vi "OCV Histogram gRPC.vi"() -> (1 "mean values of channels":dbl[](array[numeric]), 2 "std dev":dbl, 3 "range":dbl)   [LabVIEW 2019] (continued)
"battery10voltage"=0.0, "battery11voltage"=0.0, "battery12voltage"=0.0, "battery13voltage"=0.0, "battery14voltage"=0.0, "battery15voltage"=0.0, "battery16voltage"=0.0, "battery17voltage"=0.0, "battery18voltage"=0.0, "battery19voltage"=0.0, "battery20voltage"=0.0, "battery21voltage"=0.0, "battery22voltage"=0.0, "battery23voltage"=0.0, "battery24voltage"=0.0, "ErrorOutData"={"ErrorCode"=0, "ErrorMessage"=""}}, {"battery1voltage"=3.481647, "battery2voltage"=3.483053, "battery3voltage"=3.4783683, "battery4voltage"=3.4823787, "battery5voltage"=3.484421, "battery6voltage"=0.0, "battery7voltage"=0.0, "battery8voltage"=0.0, "battery9voltage"=0.0, "battery10voltage"=0.0, "battery11voltage"=0.0, "battery12voltage"=0.0, "battery13voltage"=0.0, "battery14voltage"=0.0, "battery15voltage"=0.0, "battery16voltage"=0.0, "battery17voltage"=0.0, "battery18voltage"=0.0, "battery19voltage"=0.0, "battery20voltage"=0.0, "battery21voltage"=0.0, "battery22voltage"=0.0, "battery23voltage"=0.0, "battery24voltage"=0.0, "ErrorOutData"={"ErrorCode"=0, "ErrorMessage"=""}}, {"battery1voltage"=3.4816504, "battery2voltage"=3.4830518, "battery3voltage"=3.4783711, "battery4voltage"=3.4823825, "battery5voltage"=3.484416, "battery6voltage"=0.0, "battery7voltage"=0.0, "battery8voltage"=0.0, "battery9voltage"=0.0, "battery10voltage"=0.0, "battery11voltage"=0.0, "battery12voltage"=0.0, "battery13voltage"=0.0, "battery14voltage"=0.0, "battery15voltage"=0.0, "battery16voltage"=0.0, "battery17voltage"=0.0, "battery18voltage"=0.0, "battery19voltage"=0.0, "battery20voltage"=0.0, "battery21voltage"=0.0, "battery22voltage"=0.0, "battery23voltage"=0.0, "battery24voltage"=0.0, "ErrorOutData"={"ErrorCode"=0, "ErrorMessage"=""}}, {"battery1voltage"=3.4816463, "battery2voltage"=3.483057, "battery3voltage"=3.4783702, "battery4voltage"=3.4823778, "battery5voltage"=3.4844162, "battery6voltage"=0.0, "battery7voltage"=0.0, "battery8voltage"=0.0, "battery9voltage"=0.0, "battery10voltage"=0.0, "battery11voltage"=0.0, "battery12voltage"=0.0, "battery13voltage"=0.0, "battery14voltage"=0.0, "battery15voltage"=0.0, "battery16voltage"=0.0, "battery17voltage"=0.0, "battery18voltage"=0.0, "battery19voltage"=0.0, "battery20voltage"=0.0, "battery21voltage"=0.0, "battery22voltage"=0.0, "battery23voltage"=0.0, "battery24voltage"=0.0, "ErrorOutData"={"ErrorCode"=0, "ErrorMessage"=""}}, {"battery1voltage"=3.4816453, "battery2voltage"=3.4830477, "battery3voltage"=3.4783695, "battery4voltage"=3.4823759, "battery5voltage"=3.484422, "battery6voltage"=0.0, "battery7voltage"=0.0, "battery8voltage"=0.0, "battery9voltage"=0.0, "battery10voltage"=0.0, "battery11voltage"=0.0, "battery12voltage"=0.0, "battery13voltage"=0.0, "battery14voltage"=0.0, "battery15voltage"=0.0, "battery16voltage"=0.0, "battery17voltage"=0.0, "battery18voltage"=0.0, "battery19voltage"=0.0, "battery20voltage"=0.0, "battery21voltage"=0.0, "battery22voltage"=0.0, "battery23voltage"=0.0, "battery24voltage"=0.0, "ErrorOutData"={"ErrorCode"=0, "ErrorMessage"=""}}, {"battery1voltage"=3.4816494, "battery2voltage"=3.4830532, "battery3voltage"=3.4783733, "battery4voltage"=3.4823766, "battery5voltage"=3.484416, "battery6voltage"=0.0, "battery7voltage"=0.0, "battery8voltage"=0.0, "battery9voltage"=0.0, "battery10voltage"=0.0, "battery11voltage"=0.0, "battery12voltage"=0.0, "battery13voltage"=0.0, "battery14voltage"=0.0, "battery15voltage"=0.0, "battery16voltage"=0.0, "battery17voltage"=0.0, "battery18voltage"=0.0, "battery19voltage"=0.0, "battery20voltage"=0.0, "battery21voltage"=0.0, "battery22voltage"=0.0, "battery23voltage"=0.0, "battery24voltage"=0.0, "ErrorOutData"={"ErrorCode"=0, "ErrorMessage"=""}}, {"battery1voltage"=3.4816468, "battery2voltage"=3.4830523, "battery3voltage"=3.4783683, "battery4voltage"=3.4823766, "battery5voltage"=3.4844196, "battery6voltage"=0.0, "battery7voltage"=0.0, "battery8voltage"=0.0, "battery9voltage"=0.0, "battery10voltage"=0.0, "battery11voltage"=0.0, "battery12voltage"=0.0, "battery13voltage"=0.0, "battery14voltage"=0.0, "battery15voltage"=0.0, "battery16voltage"=0.0, "battery17voltage"=0.0, "battery18voltage"=0.0, "battery19voltage"=0.0, "battery20voltage"=0.0, "battery21voltage"=0.0, "battery22voltage"=0.0, "battery23voltage"=0.0, "battery24voltage"=0.0, "ErrorOutData"={"ErrorCode"=0, "ErrorMessage"=""}}, {"battery1voltage"=3.4816508, "battery2voltage"=3.4830527, "battery3voltage"=3.4783697, "battery4voltage"=3.4823782, "battery5voltage"=3.4844193, "battery6voltage"=0.0, "battery7voltage"=0.0, "battery8voltage"=0.0, "battery9voltage"=0.0, "battery10voltage"=0.0, "battery11voltage"=0.0, "battery12voltage"=0.0, "battery13voltage"=0.0, "battery14voltage"=0.0, "battery15voltage"=0.0, "battery16voltage"=0.0, "battery17voltage"=0.0, "battery18voltage"=0.0, "battery19voltage"=0.0, "battery20voltage"=0.0, "battery21voltage"=0.0, "battery22voltage"=0.0, "battery23voltage"=0.0, "battery24voltage"=0.0, "ErrorOutData"={"ErrorCode"=0, "ErrorMessage"=""}}, {"battery1voltage"=3.481642, "battery2voltage"=3.4830513, "battery3voltage"=3.4783704, "battery4voltage"=3.4823792, "battery5voltage"=3.48442, "battery6voltage"=0.0, "battery7voltage"=0.0, "battery8voltage"=0.0, "battery9voltage"=0.0, "battery10voltage"=0.0, "battery11voltage"=0.0, "battery12voltage"=0.0, "battery13voltage"=0.0, "battery14voltage"=0.0, "battery15voltage"=0.0, "battery16voltage"=0.0, "battery17voltage"=0.0, "battery18voltage"=0.0, "battery19voltage"=0.0, "battery20voltage"=0.0, "battery21voltage"=0.0, "battery22voltage"=0.0, "battery23voltage"=0.0, "battery24voltage"=0.0, "ErrorOutData"={"ErrorCode"=0, "ErrorMessage"=""}}, {"battery1voltage"=3.4816487, "battery2voltage"=3.4830544, "battery3voltage"=3.4783728, "battery4voltage"=3.4823782, "battery5voltage"=3.4844177, "battery6voltage"=0.0, "battery7voltage"=0.0, "battery8voltage"=0.0, "battery9voltage"=0.0, "battery10voltage"=0.0, "battery11voltage"=0.0, "battery12voltage"=0.0, "battery13voltage"=0.0, "battery14voltage"=0.0, "battery15voltage"=0.0, "battery16voltage"=0.0, "battery17voltage"=0.0, "battery18voltage"=0.0, "battery19voltage"=0.0, "battery20voltage"=0.0, "battery21voltage"=0.0, "battery22voltage"=0.0, "battery23voltage"=0.0, "battery24voltage"=0.0, "ErrorOutData"={"ErrorCode"=0, "ErrorMessage"=""}}, {"battery1voltage"=3.4816446, "battery2voltage"=3.4830532, "battery3voltage"=3.478369, "battery4voltage"=3.48238, "battery5voltage"=3.4844236, "battery6voltage"=0.0, "battery7voltage"=0.0, "battery8voltage"=0.0, "battery9voltage"=0.0, "battery10voltage"=0.0, "battery11voltage"=0.0, "battery12voltage"=0.0, "battery13voltage"=0.0, "battery14voltage"=0.0, "battery15voltage"=0.0, "battery16voltage"=0.0, "battery17voltage"=0.0, "battery18voltage"=0.0, "battery19voltage"=0.0, "battery20voltage"=0.0, "battery21voltage"=0.0, "battery22voltage"=0.0, "battery23voltage"=0.0, "battery24voltage"=0.0, "ErrorOutData"={"ErrorCode"=0, "ErrorMessage"=""}}, {"battery1voltage"=3.4816463, "battery2voltage"=3.4830544, "battery3voltage"=3.4783685, "battery4voltage"=3.4823768, "battery5voltage"=3.4844203, "battery6voltage"=0.0, "battery7voltage"=0.0, "battery8voltage"=0.0, "battery9voltage"=0.0, "battery10voltage"=0.0, "battery11voltage"=0.0, "battery12voltage"=0.0, "battery13voltage"=0.0, "battery14voltage"=0.0, "battery15voltage"=0.0, "battery16voltage"=0.0, "battery17voltage"=0.0, "battery18voltage"=0.0, "battery19voltage"=0.0, "battery20voltage"=0.0, "battery21voltage"=0.0, "battery22voltage"=0.0, "battery23voltage"=0.0, "battery24voltage"=0.0, "ErrorOutData"={"ErrorCode"=0, "ErrorMessage"=""}}, {"battery1voltage"=3.4816487, "battery2voltage"=3.4830546, "battery3voltage"=3.478372, "battery4voltage"=3.4823773, "battery5voltage"=3.4844177, "battery6voltage"=0.0, "battery7voltage"=0.0, "battery8voltage"=0.0, "battery9voltage"=0.0, "battery10voltage"=0.0, "battery11voltage"=0.0, "battery12voltage"=0.0, "battery13voltage"=0.0, "battery14voltage"=0.0, "battery15voltage"=0.0, "battery16voltage"=0.0, "battery17voltage"=0.0, "battery18voltage"=0.0, "battery19voltage"=0.0, "battery20voltage"=0.0, "battery21voltage"=0.0, "battery22voltage"=0.0, "battery23voltage"=0.0, "battery24voltage"=0.0, "ErrorOutData"={"ErrorCode"=0, "ErrorMessage"=""}}, {"battery1voltage"=3.481645, "battery2voltage"=3.483051, "battery3voltage"=3.4783678, "battery4voltage"=3.4823775, "battery5voltage"=3.4844215, "battery6voltage"=0.0, "battery7voltage"=0.0, "battery8voltage"=0.0, "battery9voltage"=0.0, "battery10voltage"=0.0, "battery11voltage"=0.0, "battery12voltage"=0.0, "battery13voltage"=0.0, "battery14voltage"=0.0, "battery15voltage"=0.0, "battery16voltage"=0.0, "battery17voltage"=0.0, "battery18voltage"=0.0, "battery19voltage"=0.0, "battery20voltage"=0.0, "battery21voltage"=0.0, "battery22voltage"=0.0, "battery23voltage"=0.0, "battery24voltage"=0.0, "ErrorOutData"={"ErrorCode"=0, "ErrorMessage"=""}}, {"battery1voltage"=3.481644, "battery2voltage"=3.4830499, "battery3voltage"=3.478368, "battery4voltage"=3.4823766, "battery5voltage"=3.48442, "battery6voltage"=0.0, "battery7voltage"=0.0, "battery8voltage"=0.0, "battery9voltage"=0.0, "battery10voltage"=0.0, "battery11voltage"=0.0, "battery12voltage"=0.0, "battery13voltage"=0.0, "battery14voltage"=0.0, "battery15voltage"=0.0, "battery16voltage"=0.0, "battery17voltage"=0.0, "battery18voltage"=0.0, "battery19voltage"=0.0, "battery20voltage"=0.0, "battery21voltage"=0.0, "battery22voltage"=0.0, "battery23voltage"=0.0, "battery24voltage"=0.0, "ErrorOutData"={"ErrorCode"=0, "ErrorMessage"=""}}, {"battery1voltage"=3.4816465, "battery2voltage"=3.4830527, "battery3voltage"=3.4783714, "battery4voltage"=3.4823806, "battery5voltage"=3.4844224, "battery6voltage"=0.0, "battery7voltage"=0.0, "battery8voltage"=0.0, "battery9voltage"=0.0, "battery10voltage"=0.0, "battery11voltage"=0.0, "battery12voltage"=0.0, "battery13voltage"=0.0, "battery14voltage"=0.0, "battery15voltage"=0.0, "battery16voltage"=0.0, "battery17voltage"=0.0, "battery18voltage"=0.0, "battery19voltage"=0.0, "battery20voltage"=0.0, "battery21voltage"=0.0, "battery22voltage"=0.0, "battery23voltage"=0.0, "battery24voltage"=0.0, "ErrorOutData"={"ErrorCode"=0, "ErrorMessage"=""}}, {"battery1voltage"=3.4816434, "battery2voltage"=3.4830525, "battery3voltage"=3.478371, "battery4voltage"=3.4823768, "battery5voltage"=3.4844205, "battery6voltage"=0.0, "battery7voltage"=0.0, "battery8voltage"=0.0, "battery9voltage"=0.0, "battery10voltage"=0.0, "battery11voltage"=0.0, "battery12voltage"=0.0, "battery13voltage"=0.0, "battery14voltage"=0.0, "battery15voltage"=0.0, "battery16voltage"=0.0, "battery17voltage"=0.0, "battery18voltage"=0.0, "battery19voltage"=0.0, "battery20voltage"=0.0, "battery21voltage"=0.0, "battery22voltage"=0.0, "battery23voltage"=0.0, "battery24voltage"=0.0, "ErrorOutData"={"ErrorCode"=0, "ErrorMessage"=""}}, {"battery1voltage"=3.48165, "battery2voltage"=3.4830544, "battery3voltage"=3.478374, "battery4voltage"=3.48238, "battery5voltage"=3.484415, "battery6voltage"=0.0, "battery7voltage"=0.0, "battery8voltage"=0.0, "battery9voltage"=0.0, "battery10voltage"=0.0, "battery11voltage"=0.0, "battery12voltage"=0.0, "battery13voltage"=0.0, "battery14voltage"=0.0, "battery15voltage"=0.0, "battery16voltage"=0.0, "battery17voltage"=0.0, "battery18voltage"=0.0, "battery19voltage"=0.0, "battery20voltage"=0.0, "battery21voltage"=0.0, "battery22voltage"=0.0, "battery23voltage"=0.0, "battery24voltage"=0.0, "ErrorOutData"={"ErrorCode"=0, "ErrorMessage"=""}}, {"battery1voltage"=3.4816496, "battery2voltage"=3.4830534, "battery3voltage"=3.4783719, "battery4voltage"=3.4823778, "battery5voltage"=3.4844134, "battery6voltage"=0.0, "battery7voltage"=0.0, "battery8voltage"=0.0, "battery9voltage"=0.0, "battery10voltage"=0.0, "battery11voltage"=0.0, "battery12voltage"=0.0, "battery13voltage"=0.0, "battery14voltage"=0.0, "battery15voltage"=0.0, "battery16voltage"=0.0, "battery17voltage"=0.0, "battery18voltage"=0.0, "battery19voltage"=0.0, "battery20voltage"=0.0, "battery21voltage"=0.0, "battery22voltage"=0.0, "battery23voltage"=0.0, "battery24voltage"=0.0, "ErrorOutData"={"ErrorCode"=0, "ErrorMessage"=""}}, {"battery1voltage"=3.4816484, "battery2voltage"=3.483056, "battery3voltage"=3.478373, "battery4voltage"=3.4823804, "battery5voltage"=3.4844162, "battery6voltage"=0.0, "battery7voltage"=0.0, "battery8voltage"=0.0, "battery9voltage"=0.0, "battery10voltage"=0.0, "battery11voltage"=0.0, "battery12voltage"=0.0, "battery13voltage"=0.0, "battery14voltage"=0.0, "battery15voltage"=0.0, "battery16voltage"=0.0, "battery17voltage"=0.0, "battery18voltage"=0.0, "battery19voltage"=0.0, "battery20voltage"=0.0, "battery21voltage"=0.0, "battery22voltage"=0.0, "battery23voltage"=0.0, "battery24voltage"=0.0, "ErrorOutData"={"ErrorCode"=0, "ErrorMessage"=""}}, {"battery1voltage"=3.481651, "battery2voltage"=3.4830542, "battery3voltage"=3.4783747, "battery4voltage"=3.4823802, "battery5voltage"=3.484418, "battery6voltage"=0.0, "battery7voltage"=0.0, "battery8voltage"=0.0, "battery9voltage"=0.0, "battery10voltage"=0.0, "battery11voltage"=0.0, "battery12voltage"=0.0, "battery13voltage"=0.0, "battery14voltage"=0.0, "battery15voltage"=0.0, "battery16voltage"=0.0, "battery17voltage"=0.0, "battery18voltage"=0.0, "battery19voltage"=0.0, "battery20voltage"=0.0, "battery21voltage"=0.0, "battery22voltage"=0.0, "battery23voltage"=0.0, "battery24voltage"=0.0, "ErrorOutData"={"ErrorCode"=0, "ErrorMessage"=""}}, {"battery1voltage"=3.4816492, "battery2voltage"=3.4830544, "battery3voltage"=3.4783723, "battery4voltage"=3.4823797, "battery5voltage"=3.484417, "battery6voltage"=0.0, "battery7voltage"=0.0, "battery8voltage"=0.0, "battery9voltage"=0.0, "battery10voltage"=0.0, "battery11voltage"=0.0, "battery12voltage"=0.0, "battery13voltage"=0.0, "battery14voltage"=0.0, "battery15voltage"=0.0, "battery16voltage"=0.0, "battery17voltage"=0.0, "battery18voltage"=0.0, "battery19voltage"=0.0, "battery20voltage"=0.0, "battery21voltage"=0.0, "battery22voltage"=0.0, "battery23voltage"=0.0, "battery24voltage"=0.0, "ErrorOutData"={"ErrorCode"=0, "ErrorMessage"=""}}, {"battery1voltage"=3.481646, "battery2voltage"=3.483055, "battery3voltage"=3.4783723, "battery4voltage"=3.4823785, "battery5voltage"=3.4844184, "battery6voltage"=0.0, "battery7voltage"=0.0, "battery8voltage"=0.0, "battery9voltage"=0.0, "battery10voltage"=0.0, "battery11voltage"=0.0, "battery12voltage"=0.0, "battery13voltage"=0.0, "battery14voltage"=0.0, "battery15voltage"=0.0, "battery16voltage"=0.0, "battery17voltage"=0.0, "battery18voltage"=0.0, "battery19voltage"=0.0, "battery20voltage"=0.0, "battery21voltage"=0.0, "battery22voltage"=0.0, "battery23voltage"=0.0, "battery24voltage"=0.0, "ErrorOutData"={"ErrorCode"=0, "ErrorMessage"=""}}, {"battery1voltage"=3.4816487, "battery2voltage"=3.483054, "battery3voltage"=3.478376, "battery4voltage"=3.482378, "battery5voltage"=3.4844177, "battery6voltage"=0.0, "battery7voltage"=0.0, "battery8voltage"=0.0, "battery9voltage"=0.0, "battery10voltage"=0.0, "battery11voltage"=0.0, "battery12voltage"=0.0, "battery13voltage"=0.0, "battery14voltage"=0.0, "battery15voltage"=0.0, "battery16voltage"=0.0, "battery17voltage"=0.0, "battery18voltage"=0.0, "battery19voltage"=0.0, "battery20voltage"=0.0, "battery21voltage"=0.0, "battery22voltage"=0.0, "battery23voltage"=0.0, "battery24voltage"=0.0, "ErrorOutData"={"ErrorCode"=0, "ErrorMessage"=""}}, {"battery1voltage"=3.481652, "battery2voltage"=3.483055, "battery3voltage"=3.4783716, "battery4voltage"=3.4823794, "battery5voltage"=3.4844162, "battery6voltage"=0.0, "battery7voltage"=0.0, "battery8voltage"=0.0, "battery9voltage"=0.0, "battery10voltage"=0.0, "battery11voltage"=0.0, "battery12voltage"=0.0, "battery13voltage"=0.0, "battery14voltage"=0.0, "battery15voltage"=0.0, "battery16voltage"=0.0, "battery17voltage"=0.0, "battery18voltage"=0.0, "battery19voltage"=0.0, "battery20voltage"=0.0, "battery21voltage"=0.0, "battery22voltage"=0.0, "battery23voltage"=0.0, "battery24voltage"=0.0, "ErrorOutData"={"ErrorCode"=0, "ErrorMessage"=""}}, {"battery1voltage"=3.4816456, "battery2voltage"=3.4830518, "battery3voltage"=3.4783688, "battery4voltage"=3.4823813, "battery5voltage"=3.4844205, "battery6voltage"=0.0, "battery7voltage"=0.0, "battery8voltage"=0.0, "battery9voltage"=0.0, "battery10voltage"=0.0, "battery11voltage"=0.0, "battery12voltage"=0.0, "battery13voltage"=0.0, "battery14voltage"=0.0, "battery15voltage"=0.0, "battery16voltage"=0.0, "battery17voltage"=0.0, "battery18voltage"=0.0, "battery19voltage"=0.0, "battery20voltage"=0.0, "battery21voltage"=0.0, "battery22voltage"=0.0, "battery23voltage"=0.0, "battery24voltage"=0.0, "ErrorOutData"={"ErrorCode"=0, "ErrorMessage"=""}}, {"battery1voltage"=3.4816494, "battery2voltage"=3.4830585, "battery3voltage"=3.478372, "battery4voltage"=3.4823797, "battery5voltage"=3.48442, "battery6voltage"=0.0, "battery7voltage"=0.0, "battery8voltage"=0.0, "battery9voltage"=0.0, "battery10voltage"=0.0, "battery11voltage"=0.0, "battery12voltage"=0.0, "battery13voltage"=0.0, "battery14voltage"=0.0, "battery15voltage"=0.0, "battery16voltage"=0.0, "battery17voltage"=0.0, "battery18voltage"=0.0, "battery19voltage"=0.0, "battery20voltage"=0.0, "battery21voltage"=0.0, "battery22voltage"=0.0, "battery23voltage"=0.0, "battery24voltage"=0.0, "ErrorOutData"={"ErrorCode"=0, "ErrorMessage"=""}}, {"battery1voltage"=3.481647, "battery2voltage"=3.483051, "battery3voltage"=3.478373, "battery4voltage"=3.4823787, "battery5voltage"=3.484418, "battery6voltage"=0.0, "battery7voltage"=0.0, "battery8voltage"=0.0, "battery9voltage"=0.0, "battery10voltage"=0.0, "battery11voltage"=0.0, "battery12voltage"=0.0, "battery13voltage"=0.0, "battery14voltage"=0.0, "battery15voltage"=0.0, "battery16voltage"=0.0, "battery17voltage"=0.0, "battery18voltage"=0.0, "battery19voltage"=0.0, "battery20voltage"=0.0, "battery21voltage"=0.0, "battery22voltage"=0.0, "battery23voltage"=0.0, "battery24voltage"=0.0, "ErrorOutData"={"ErrorCode"=0, "ErrorMessage"=""}}, {"battery1voltage"=3.4816463, "battery2voltage"=3.4830534, "battery3voltage"=3.4783728, "battery4voltage"=3.4823809, "battery5voltage"=3.484416, "battery6voltage"=0.0, "battery7voltage"=0.0, "battery8voltage"=0.0, "battery9voltage"=0.0, "battery10voltage"=0.0, "battery11voltage"=0.0, "battery12voltage"=0.0, "battery13voltage"=0.0, "battery14voltage"=0.0, "battery15voltage"=0.0, "battery16voltage"=0.0, "battery17voltage"=0.0, "battery18voltage"=0.0, "battery19voltage"=0.0, "battery20voltage"=0.0, "battery21voltage"=0.0, "battery22voltage"=0.0, "battery23voltage"=0.0, "battery24voltage"=0.0, "ErrorOutData"={"ErrorCode"=0, "ErrorMessage"=""}}, {"battery1voltage"=3.4816506, "battery2voltage"=3.4830523, "battery3voltage"=3.4783754, "battery4voltage"=3.48238, "battery5voltage"=3.4844172, "battery6voltage"=0.0, "battery7voltage"=0.0, "battery8voltage"=0.0, "battery9voltage"=0.0, "battery10voltage"=0.0, "battery11voltage"=0.0, "battery12voltage"=0.0, "battery13voltage"=0.0, "battery14voltage"=0.0, "battery15voltage"=0.0, "battery16voltage"=0.0, "battery17voltage"=0.0, "battery18voltage"=0.0, "battery19voltage"=0.0, "battery20voltage"=0.0, "battery21voltage"=0.0, "battery22voltage"=0.0, "battery23voltage"=0.0, "battery24voltage"=0.0, "ErrorOutData"={"ErrorCode"=0, "ErrorMessage"=""}}, {"battery1voltage"=3.481645, "battery2voltage"=3.4830508, "battery3voltage"=3.4783704, "battery4voltage"=3.4823787, "battery5voltage"=3.4844234, "battery6voltage"=0.0, "battery7voltage"=0.0, "battery8voltage"=0.0, "battery9voltage"=0.0, "battery10voltage"=0.0, "battery11voltage"=0.0, "battery12voltage"=0.0, "battery13voltage"=0.0, "battery14voltage"=0.0, "battery15voltage"=0.0, "battery16voltage"=0.0, "battery17voltage"=0.0, "battery18voltage"=0.0, "battery19voltage"=0.0, "battery20voltage"=0.0, "battery21voltage"=0.0, "battery22voltage"=0.0, "battery23voltage"=0.0, "battery24voltage"=0.0, "ErrorOutData"={"ErrorCode"=0, "ErrorMessage"=""}}, {"battery1voltage"=3.4816458, "battery2voltage"=3.4830515, "battery3voltage"=3.4783695, "battery4voltage"=3.4823802, "battery5voltage"=3.4844224, "battery6voltage"=0.0, "battery7voltage"=0.0, "battery8voltage"=0.0, "battery9voltage"=0.0, "battery10voltage"=0.0, "battery11voltage"=0.0, "battery12voltage"=0.0, "battery13voltage"=0.0, "battery14voltage"=0.0, "battery15voltage"=0.0, "battery16voltage"=0.0, "battery17voltage"=0.0, "battery18voltage"=0.0, "battery19voltage"=0.0, "battery20voltage"=0.0, "battery21voltage"=0.0, "battery22voltage"=0.0, "battery23voltage"=0.0, "battery24voltage"=0.0, "ErrorOutData"={"ErrorCode"=0, "ErrorMessage"=""}}, {"battery1voltage"=3.4816506, "battery2voltage"=3.4830563, "battery3voltage"=3.4783714, "battery4voltage"=3.4823754, "battery5voltage"=3.48442, "battery6voltage"=0.0, "battery7voltage"=0.0, "battery8voltage"=0.0, "battery9voltage"=0.0, "battery10voltage"=0.0, "battery11voltage"=0.0, "battery12voltage"=0.0, "battery13voltage"=0.0, "battery14voltage"=0.0, "battery15voltage"=0.0, "battery16voltage"=0.0, "battery17voltage"=0.0, "battery18voltage"=0.0, "battery19voltage"=0.0, "battery20voltage"=0.0, "battery21voltage"=0.0, "battery22voltage"=0.0, "battery23voltage"=0.0, "battery24voltage"=0.0, "ErrorOutData"={"ErrorCode"=0, "ErrorMessage"=""}}, {"battery1voltage"=3.4816504, "battery2voltage"=3.483054, "battery3voltage"=3.4783735, "battery4voltage"=3.4823773, "battery5voltage"=3.4844174, "battery6voltage"=0.0, "battery7voltage"=0.0, "battery8voltage"=0.0, "battery9voltage"=0.0, "battery10voltage"=0.0, "battery11voltage"=0.0, "battery12voltage"=0.0, "battery13voltage"=0.0, "battery14voltage"=0.0, "battery15voltage"=0.0, "battery16voltage"=0.0, "battery17voltage"=0.0, "battery18voltage"=0.0, "battery19voltage"=0.0, "battery20voltage"=0.0, "battery21voltage"=0.0, "battery22voltage"=0.0, "battery23voltage"=0.0, "battery24voltage"=0.0, "ErrorOutData"={"ErrorCode"=0, "ErrorMessage"=""}}, {"battery1voltage"=3.4816496, "battery2voltage"=3.4830523, "battery3voltage"=3.4783714, "battery4voltage"=3.482379, "battery5voltage"=3.4844172, "battery6voltage"=0.0, "battery7voltage"=0.0, "battery8voltage"=0.0, "battery9voltage"=0.0, "battery10voltage"=0.0, "battery11voltage"=0.0, "battery12voltage"=0.0, "battery13voltage"=0.0, "battery14voltage"=0.0, "battery15voltage"=0.0, "battery16voltage"=0.0, "battery17voltage"=0.0, "battery18voltage"=0.0, "battery19voltage"=0.0, "battery20voltage"=0.0, "battery21voltage"=0.0, "battery22voltage"=0.0, "battery23voltage"=0.0, "battery24voltage"=0.0, "ErrorOutData"={"ErrorCode"=0, "ErrorMessage"=""}}, {"battery1voltage"=3.4816484, "battery2voltage"=3.4830527, "battery3voltage"=3.4783726, "battery4voltage"=3.4823809, "battery5voltage"=3.4844155, "battery6voltage"=0.0, "battery7voltage"=0.0, "battery8voltage"=0.0, "battery9voltage"=0.0, "battery10voltage"=0.0, "battery11voltage"=0.0, "battery12voltage"=0.0, "battery13voltage"=0.0, "battery14voltage"=0.0, "battery15voltage"=0.0, "battery16voltage"=0.0, "battery17voltage"=0.0, "battery18voltage"=0.0, "battery19voltage"=0.0, "battery20voltage"=0.0, "battery21voltage"=0.0, "battery22voltage"=0.0, "battery23voltage"=0.0, "battery24voltage"=0.0, "ErrorOutData"={"ErrorCode"=0, "ErrorMessage"=""}}, {"battery1voltage"=3.4816446, "battery2voltage"=3.4830515, "battery3voltage"=3.4783666, "battery4voltage"=3.4823778, "battery5voltage"=3.4844198, "battery6voltage"=0.0, "battery7voltage"=0.0, "battery8voltage"=0.0, "battery9voltage"=0.0, "battery10voltage"=0.0, "battery11voltage"=0.0, "battery12voltage"=0.0, "battery13voltage"=0.0, "battery14voltage"=0.0, "battery15voltage"=0.0, "battery16voltage"=0.0, "battery17voltage"=0.0, "battery18voltage"=0.0, "battery19voltage"=0.0, "battery20voltage"=0.0, "battery21voltage"=0.0, "battery22voltage"=0.0, "battery23voltage"=0.0, "battery24voltage"=0.0, "ErrorOutData"={"ErrorCode"=0, "ErrorMessage"=""}}, {"battery1voltage"=3.4816475, "battery2voltage"=3.4830492, "battery3voltage"=3.4783704, "battery4voltage"=3.482381, "battery5voltage"=3.4844236, "battery6voltage"=0.0, "battery7voltage"=0.0, "battery8voltage"=0.0, "battery9voltage"=0.0, "battery10voltage"=0.0, "battery11voltage"=0.0, "battery12voltage"=0.0, "battery13voltage"=0.0, "battery14voltage"=0.0, "battery15voltage"=0.0, "battery16voltage"=0.0, "battery17voltage"=0.0, "battery18voltage"=0.0, "battery19voltage"=0.0, "battery20voltage"=0.0, "battery21voltage"=0.0, "battery22voltage"=0.0, "battery23voltage"=0.0, "battery24voltage"=0.0, "ErrorOutData"={"ErrorCode"=0, "ErrorMessage"=""}}, {"battery1voltage"=3.481648, "battery2voltage"=3.4830556, "battery3voltage"=3.47837, "battery4voltage"=3.482381, "battery5voltage"=3.4844158, "battery6voltage"=0.0, "battery7voltage"=0.0, "battery8voltage"=0.0, "battery9voltage"=0.0, "battery10voltage"=0.0, "battery11voltage"=0.0, "battery12voltage"=0.0, "battery13voltage"=0.0, "battery14voltage"=0.0, "battery15voltage"=0.0, "battery16voltage"=0.0, "battery17voltage"=0.0, "battery18voltage"=0.0, "battery19voltage"=0.0, "battery20voltage"=0.0, "battery21voltage"=0.0, "battery22voltage"=0.0, "battery23voltage"=0.0, "battery24voltage"=0.0, "ErrorOutData"={"ErrorCode"=0, "ErrorMessage"=""}}, {"battery1voltage"=3.48165, "battery2voltage"=3.4830525, "battery3voltage"=3.478371, "battery4voltage"=3.4823828, "battery5voltage"=3.4844155, "battery6voltage"=0.0, "battery7voltage"=0.0, "battery8voltage"=0.0, "battery9voltage"=0.0, "battery10voltage"=0.0, "battery11voltage"=0.0, "battery12voltage"=0.0, "battery13voltage"=0.0, "battery14voltage"=0.0, "battery15voltage"=0.0, "battery16voltage"=0.0, "battery17voltage"=0.0, "battery18voltage"=0.0, "battery19voltage"=0.0, "battery20voltage"=0.0, "battery21voltage"=0.0, "battery22voltage"=0.0, "battery23voltage"=0.0, "battery24voltage"=0.0, "ErrorOutData"={"ErrorCode"=0, "ErrorMessage"=""}}, {"battery1voltage"=3.4816492, "battery2voltage"=3.4830534, "battery3voltage"=3.4783719, "battery4voltage"=3.4823785, "battery5voltage"=3.484423, "battery6voltage"=0.0, "battery7voltage"=0.0, "battery8voltage"=0.0, "battery9voltage"=0.0, "battery10voltage"=0.0, "battery11voltage"=0.0, "battery12voltage"=0.0, "battery13voltage"=0.0, "battery14voltage"=0.0, "battery15voltage"=0.0, "battery16voltage"=0.0, "battery17voltage"=0.0, "battery18voltage"=0.0, "battery19voltage"=0.0, "battery20voltage"=0.0, "battery21voltage"=0.0, "battery22voltage"=0.0, "battery23voltage"=0.0, "battery24voltage"=0.0, "ErrorOutData"={"ErrorCode"=0, "ErrorMessage"=""}}, {"battery1voltage"=3.481646, "battery2voltage"=3.483051, "battery3voltage"=3.478368, "battery4voltage"=3.4823785, "battery5voltage"=3.4844213, "battery6voltage"=0.0, "battery7voltage"=0.0, "battery8voltage"=0.0, "battery9voltage"=0.0, "battery10voltage"=0.0, "battery11voltage"=0.0, "battery12voltage"=0.0, "battery13voltage"=0.0, "battery14voltage"=0.0, "battery15voltage"=0.0, "battery16voltage"=0.0, "battery17voltage"=0.0, "battery18voltage"=0.0, "battery19voltage"=0.0, "battery20voltage"=0.0, "battery21voltage"=0.0, "battery22voltage"=0.0, "battery23voltage"=0.0, "battery24voltage"=0.0, "ErrorOutData"={"ErrorCode"=0, "ErrorMessage"=""}}, {"battery1voltage"=3.4816432, "battery2voltage"=3.4830525, "battery3voltage"=3.4783711, "battery4voltage"=3.4823782, "battery5voltage"=3.484421, "battery6voltage"=0.0, "battery7voltage"=0.0, "battery8voltage"=0.0, "battery9voltage"=0.0, "battery10voltage"=0.0, "battery11voltage"=0.0, "battery12voltage"=0.0, "battery13voltage"=0.0, "battery14voltage"=0.0, "battery15voltage"=0.0, "battery16voltage"=0.0, "battery17voltage"=0.0, "battery18voltage"=0.0, "battery19voltage"=0.0, "battery20voltage"=0.0, "battery21voltage"=0.0, "battery22voltage"=0.0, "battery23voltage"=0.0, "battery24voltage"=0.0, "ErrorOutData"={"ErrorCode"=0, "ErrorMessage"=""}}, {"battery1voltage"=3.481647, "battery2voltage"=3.4830503, "battery3voltage"=3.4783683, "battery4voltage"=3.4823802, "battery5voltage"=3.4844222, "battery6voltage"=0.0, "battery7voltage"=0.0, "battery8voltage"=0.0, "battery9voltage"=0.0, "battery10voltage"=0.0, "battery11voltage"=0.0, "battery12voltage"=0.0, "battery13voltage"=0.0, "battery14voltage"=0.0, "battery15voltage"=0.0, "battery16voltage"=0.0, "battery17voltage"=0.0, "battery18voltage"=0.0, "battery19voltage"=0.0, "battery20voltage"=0.0, "battery21voltage"=0.0, "battery22voltage"=0.0, "battery23voltage"=0.0, "battery24voltage"=0.0, "ErrorOutData"={"ErrorCode"=0, "ErrorMessage"=""}}, {"battery1voltage"=3.4816525, "battery2voltage"=3.4830537, "battery3voltage"=3.4783742, "battery4voltage"=3.482379, "battery5voltage"=3.4844177, "battery6voltage"=0.0, "battery7voltage"=0.0, "battery8voltage"=0.0, "battery9voltage"=0.0, "battery10voltage"=0.0, "battery11voltage"=0.0, "battery12voltage"=0.0, "battery13voltage"=0.0, "battery14voltage"=0.0, "battery15voltage"=0.0, "battery16voltage"=0.0, "battery17voltage"=0.0, "battery18voltage"=0.0, "battery19voltage"=0.0, "battery20voltage"=0.0, "battery21voltage"=0.0, "battery22voltage"=0.0, "battery23voltage"=0.0, "battery24voltage"=0.0, "ErrorOutData"={"ErrorCode"=0, "ErrorMessage"=""}}, {"battery1voltage"=3.481646, "battery2voltage"=3.4830525, "battery3voltage"=3.478367, "battery4voltage"=3.4823794, "battery5voltage"=3.484421, "battery6voltage"=0.0, "battery7voltage"=0.0, "battery8voltage"=0.0, "battery9voltage"=0.0, "battery10voltage"=0.0, "battery11voltage"=0.0, "battery12voltage"=0.0, "battery13voltage"=0.0, "battery14voltage"=0.0, "battery15voltage"=0.0, "battery16voltage"=0.0, "battery17voltage"=0.0, "battery18voltage"=0.0, "battery19voltage"=0.0, "battery20voltage"=0.0, "battery21voltage"=0.0, "battery22voltage"=0.0, "battery23voltage"=0.0, "battery24voltage"=0.0, "ErrorOutData"={"ErrorCode"=0, "ErrorMessage"=""}}, {"battery1voltage"=3.4816458, "battery2voltage"=3.483057, "battery3voltage"=3.4783719, "battery4voltage"=3.4823794, "battery5voltage"=3.484418, "battery6voltage"=0.0, "battery7voltage"=0.0, "battery8voltage"=0.0, "battery9voltage"=0.0, "battery10voltage"=0.0, "battery11voltage"=0.0, "battery12voltage"=0.0, "battery13voltage"=0.0, "battery14voltage"=0.0, "battery15voltage"=0.0, "battery16voltage"=0.0, "battery17voltage"=0.0, "battery18voltage"=0.0, "battery19voltage"=0.0, "battery20voltage"=0.0, "battery21voltage"=0.0, "battery22voltage"=0.0, "battery23voltage"=0.0, "battery24voltage"=0.0, "ErrorOutData"={"ErrorCode"=0, "ErrorMessage"=""}}, {"battery1voltage"=3.481649, "battery2voltage"=3.483054, "battery3voltage"=3.4783723, "battery4voltage"=3.4823787, "battery5voltage"=3.4844196, "battery6voltage"=0.0, "battery7voltage"=0.0, "battery8voltage"=0.0, "battery9voltage"=0.0, "battery10voltage"=0.0, "battery11voltage"=0.0, "battery12voltage"=0.0, "battery13voltage"=0.0, "battery14voltage"=0.0, "battery15voltage"=0.0, "battery16voltage"=0.0, "battery17voltage"=0.0, "battery18voltage"=0.0, "battery19voltage"=0.0, "battery20voltage"=0.0, "battery21voltage"=0.0, "battery22voltage"=0.0, "battery23voltage"=0.0, "battery24voltage"=0.0, "ErrorOutData"={"ErrorCode"=0, "ErrorMessage"=""}}, {"battery1voltage"=3.4816475, "battery2voltage"=3.4830508, "battery3voltage"=3.4783697, "battery4voltage"=3.4823792, "battery5voltage"=3.4844222, "battery6voltage"=0.0, "battery7voltage"=0.0, "battery8voltage"=0.0, "battery9voltage"=0.0, "battery10voltage"=0.0, "battery11voltage"=0.0, "battery12voltage"=0.0, "battery13voltage"=0.0, "battery14voltage"=0.0, "battery15voltage"=0.0, "battery16voltage"=0.0, "battery17voltage"=0.0, "battery18voltage"=0.0, "battery19voltage"=0.0, "battery20voltage"=0.0, "battery21voltage"=0.0, "battery22voltage"=0.0, "battery23voltage"=0.0, "battery24voltage"=0.0, "ErrorOutData"={"ErrorCode"=0, "ErrorMessage"=""}}, {"battery1voltage"=3.4816527, "battery2voltage"=3.4830518, "battery3voltage"=3.4783738, "battery4voltage"=3.482376, "battery5voltage"=3.4844162, "battery6voltage"=0.0, "battery7voltage"=0.0, "battery8voltage"=0.0, "battery9voltage"=0.0, "battery10voltage"=0.0, "battery11voltage"=0.0, "battery12voltage"=0.0, "battery13voltage"=0.0, "battery14voltage"=0.0, "battery15voltage"=0.0, "battery16voltage"=0.0, "battery17voltage"=0.0, "battery18voltage"=0.0, "battery19voltage"=0.0, "battery20voltage"=0.0, "battery21voltage"=0.0, "battery22voltage"=0.0, "battery23voltage"=0.0, "battery24voltage"=0.0, "ErrorOutData"={"ErrorCode"=0, "ErrorMessage"=""}}, {"battery1voltage"=3.4816487, "battery2voltage"=3.4830534, "battery3voltage"=3.4783742, "battery4voltage"=3.4823773, "battery5voltage"=3.4844174, "battery6voltage"=0.0, "battery7voltage"=0.0, "battery8voltage"=0.0, "battery9voltage"=0.0, "battery10voltage"=0.0, "battery11voltage"=0.0, "battery12voltage"=0.0, "battery13voltage"=0.0, "battery14voltage"=0.0, "battery15voltage"=0.0, "battery16voltage"=0.0, "battery17voltage"=0.0, "battery18voltage"=0.0, "battery19voltage"=0.0, "battery20voltage"=0.0, "battery21voltage"=0.0, "battery22voltage"=0.0, "battery23voltage"=0.0, "battery24voltage"=0.0, "ErrorOutData"={"ErrorCode"=0, "ErrorMessage"=""}}, {"battery1voltage"=3.4816446, "battery2voltage"=3.4830534, "battery3voltage"=3.47837, "battery4voltage"=3.4823787, "battery5voltage"=3.4844232, "battery6voltage"=0.0, "battery7voltage"=0.0, "battery8voltage"=0.0, "battery9voltage"=0.0, "battery10voltage"=0.0, "battery11voltage"=0.0, "battery12voltage"=0.0, "battery13voltage"=0.0, "battery14voltage"=0.0, "battery15voltage"=0.0, "battery16voltage"=0.0, "battery17voltage"=0.0, "battery18voltage"=0.0, "battery19voltage"=0.0, "battery20voltage"=0.0, "battery21voltage"=0.0, "battery22voltage"=0.0, "battery23voltage"=0.0, "battery24voltage"=0.0, "ErrorOutData"={"ErrorCode"=0, "ErrorMessage"=""}}, {"battery1voltage"=3.4816446, "battery2voltage"=3.4830508, "battery3voltage"=3.47837, "battery4voltage"=3.4823792, "battery5voltage"=3.4844208, "battery6voltage"=0.0, "battery7voltage"=0.0, "battery8voltage"=0.0, "battery9voltage"=0.0, "battery10voltage"=0.0, "battery11voltage"=0.0, "battery12voltage"=0.0, "battery13voltage"=0.0, "battery14voltage"=0.0, "battery15voltage"=0.0, "battery16voltage"=0.0, "battery17voltage"=0.0, "battery18voltage"=0.0, "battery19voltage"=0.0, "battery20voltage"=0.0, "battery21voltage"=0.0, "battery22voltage"=0.0, "battery23voltage"=0.0, "battery24voltage"=0.0, "ErrorOutData"={"ErrorCode"=0, "ErrorMessage"=""}}, {"battery1voltage"=3.4816437, "battery2voltage"=3.4830518, "battery3voltage"=3.4783685, "battery4voltage"=3.482379, "battery5voltage"=3.4844215, "battery6voltage"=0.0, "battery7voltage"=0.0, "battery8voltage"=0.0, "battery9voltage"=0.0, "battery10voltage"=0.0, "battery11voltage"=0.0, "battery12voltage"=0.0, "battery13voltage"=0.0, "battery14voltage"=0.0, "battery15voltage"=0.0, "battery16voltage"=0.0, "battery17voltage"=0.0, "battery18voltage"=0.0, "battery19voltage"=0.0, "battery20voltage"=0.0, "battery21voltage"=0.0, "battery22voltage"=0.0, "battery23voltage"=0.0, "battery24voltage"=0.0, "ErrorOutData"={"ErrorCode"=0, "ErrorMessage"=""}}, {"battery1voltage"=3.4816499, "battery2voltage"=3.483053, "battery3voltage"=3.4783704, "battery4voltage"=3.4823766, "battery5voltage"=3.484418, "battery6voltage"=0.0, "battery7voltage"=0.0, "battery8voltage"=0.0, "battery9voltage"=0.0, "battery10voltage"=0.0, "battery11voltage"=0.0, "battery12voltage"=0.0, "battery13voltage"=0.0, "battery14voltage"=0.0, "battery15voltage"=0.0, "battery16voltage"=0.0, "battery17voltage"=0.0, "battery18voltage"=0.0, "battery19voltage"=0.0, "battery20voltage"=0.0, "battery21voltage"=0.0, "battery22voltage"=0.0, "battery23voltage"=0.0, "battery24voltage"=0.0, "ErrorOutData"={"ErrorCode"=0, "ErrorMessage"=""}}, {"battery1voltage"=3.481647, "battery2voltage"=3.4830527, "battery3voltage"=3.478371, "battery4voltage"=3.4823785, "battery5voltage"=3.4844253, "battery6voltage"=0.0, "battery7voltage"=0.0, "battery8voltage"=0.0, "battery9voltage"=0.0, "battery10voltage"=0.0, "battery11voltage"=0.0, "battery12voltage"=0.0, "battery13voltage"=0.0, "battery14voltage"=0.0, "battery15voltage"=0.0, "battery16voltage"=0.0, "battery17voltage"=0.0, "battery18voltage"=0.0, "battery19voltage"=0.0, "battery20voltage"=0.0, "battery21voltage"=0.0, "battery22voltage"=0.0, "battery23voltage"=0.0, "battery24voltage"=0.0, "ErrorOutData"={"ErrorCode"=0, "ErrorMessage"=""}}]
  out "ch4 range":dbl=1.621246337890625e-05 format="%#_6p"
  out "ch4 std dev":dbl=3.4826254869466815e-06 format="%#.3p"
  out "ch4 mean":dbl=3.4844029903411866 format="%#.6p"
  out "Histogram Graph ch4":T3(graph)={"X Values"=[3.4843960762023927, 3.4843976974487307, 3.484399318695069, 3.484400939941407, 3.484402561187745, 3.484404182434083, 3.484405803680421, 3.484407424926759, 3.484409046173097, 3.4844106674194353], "Histogram: h(x)"=[5, 15, 28, 32, 24, 31, 37, 16, 8, 4]}
  out "Waveform Chart ch4":sgl[](graph)=[3.4843996, 3.4844058, 3.4844077, 3.4844036, 3.4843988, 3.4843998, 3.4844058, 3.4844072, 3.4844098, 3.4844012, 3.4844048, 3.4844062, 3.484404, 3.484405, 3.4844084, 3.4843993, 3.484403, 3.484403, 3.484405, 3.4844031, 3.4843984, 3.4844046, 3.4844067, 3.4844062, 3.4844053, 3.4844048, 3.4844077, 3.4844024, 3.484407, 3.4843976, 3.4844053, 3.4843984, 3.4844093, 3.4844065, 3.4844074, 3.4844053, 3.4843953, 3.4844062, 3.4844098, 3.4844012, 3.4844048, 3.4844093, 3.4844093, 3.4844036, 3.4844048, 3.4843988, 3.4844115, 3.4844046, 3.4844015, 3.4844108, 3.4844015, 3.4844065, 3.484401, 3.4844022, 3.4844005, 3.4844046, 3.4844015, 3.4844017, 3.4844005, 3.4844038, 3.484401, 3.4844065, 3.4844038, 3.4843976, 3.4844043, 3.4843962, 3.484406, 3.484411, 3.4844053, 3.484405, 3.4844062, 3.4844058, 3.4844027, 3.4844081, 3.4844038, 3.484406, 3.4844017, 3.4844015, 3.4844034, 3.4844112, 3.4844022, 3.4844034, 3.4844053, 3.4843974, 3.484408, 3.484399, 3.484402, 3.4843986, 3.4843988, 3.4844034, 3.4844007, 3.484406, 3.4843996, 3.484407, 3.4844058, 3.4844007, 3.4844005, 3.4844, 3.4844046, 3.4844081, 3.4844027, 3.4843986, 3.4844017, 3.4844036, 3.4843993, 3.4844043, 3.4844017, 3.4844038, 3.4844, 3.4844058, 3.4844048, 3.484407, 3.4844003, 3.4844043, 3.4844031, 3.484405, 3.4844072, 3.484408, 3.4844058, 3.4844027, 3.4843988, 3.4844024, 3.4844072, 3.4844048, 3.4844031, 3.4843996, 3.4844015, 3.4843996, 3.4844053, 3.4844053, 3.484405, 3.4844005, 3.4844043, 3.4844022, 3.4844015, 3.484406, 3.484409, 3.4843972, 3.4843993, 3.4843976, 3.484401, 3.484405, 3.4844005, 3.4844024, 3.4843972, 3.4844015, 3.4844038, 3.4843986, 3.4844007, 3.4843998, 3.4844058, 3.4844017, 3.4843976, 3.4843986, 3.4844024, 3.4844031, 3.4843988, 3.4843976, 3.4843976, 3.4844024, 3.4843974, 3.4844017, 3.4844, 3.4844055, 3.4844022, 3.4843988, 3.4843962, 3.4844062, 3.4843974, 3.484399, 3.4843974, 3.484396, 3.4844003, 3.4844074, 3.4844034, 3.484401, 3.4844058, 3.4844055, 3.4843984, 3.4843957, 3.484402, 3.4843996, 3.484405, 3.484401, 3.4844015, 3.4843998, 3.484404, 3.4844031, 3.4844012, 3.484403, 3.4843998, 3.4844034, 3.484399, 3.484402, 3.4844048, 3.484403, 3.484406, 3.4844096, 3.484407, 3.4844046]
  out "ch3 range":dbl=1.4066696166992188e-05 format="%#_6p"
  out "ch3 std dev":dbl=2.703397559171438e-06 format="%#.3p"
  out "ch3 mean":dbl=3.4823670625686645 format="%#.6p"
  out "Histogram Graph ch3":T3(graph)={"X Values"=[3.4823603510856627, 3.4823617577552795, 3.4823631644248962, 3.482364571094513, 3.48236597776413, 3.4823673844337466, 3.4823687911033634, 3.48237019777298, 3.482371604442597, 3.4823730111122138], "Histogram: h(x)"=[3, 7, 14, 30, 35, 40, 36, 19, 12, 4]}
  out "ch2 range":dbl=1.5020370483398438e-05 format="%#_6p"
  out "ch2 std dev":dbl=3.0624530062047095e-06 format="%#.3p"
  out "ch2 mean":dbl=3.478371295928955 format="%#.6p"
  out "Histogram Graph ch2":T3(graph)={"X Values"=[3.4783649802207948, 3.4783664822578433, 3.478367984294892, 3.4783694863319403, 3.478370988368989, 3.4783724904060374, 3.478373992443086, 3.4783754944801344, 3.478376996517183, 3.4783784985542314], "Histogram: h(x)"=[8, 16, 17, 38, 32, 32, 35, 10, 7, 5]}
  out "ch1 range":dbl=1.5735626220703125e-05 format="%#_6p"
  out "ch1 std dev":dbl=2.9857574743435946e-06 format="%#.3p"
  out "ch1 mean":dbl=3.4830422377586365 format="%#.6p"
  out "Histogram Graph ch1":T3(graph)={"X Values"=[3.4830358743667604, 3.4830374479293824, 3.4830390214920044, 3.4830405950546264, 3.4830421686172484, 3.4830437421798703, 3.4830453157424923, 3.4830468893051143, 3.4830484628677363, 3.4830500364303583], "Histogram: h(x)"=[4, 15, 24, 39, 37, 35, 25, 15, 5, 1]}
  out "ch0 range":dbl=1.6450881958007812e-05 format="%#_6p"
  out "ch0 std dev":dbl=2.907318571584298e-06 format="%#.3p"
  out "ch0 mean":dbl=3.4816378843784332 format="%#.6p"
  out "Histogram Graph ch0":T3(graph)={"X Values"=[3.481629478931427, 3.4816311240196227, 3.4816327691078186, 3.4816344141960145, 3.4816360592842104, 3.4816377043724063, 3.481639349460602, 3.481640994548798, 3.481642639636994, 3.48164428472519], "Histogram: h(x)"=[1, 1, 10, 26, 32, 51, 28, 39, 6, 6]}
  out "Waveform Chart ch1":sgl[](graph)=[3.4830456, 3.4830368, 3.4830387, 3.4830468, 3.4830465, 3.4830382, 3.4830444, 3.483041, 3.4830418, 3.4830396, 3.483039, 3.4830399, 3.4830463, 3.4830413, 3.4830387, 3.4830422, 3.4830387, 3.483043, 3.483041, 3.4830444, 3.4830453, 3.4830413, 3.4830446, 3.48304, 3.483041, 3.4830427, 3.4830396, 3.4830408, 3.483045, 3.483045, 3.4830372, 3.4830437, 3.4830418, 3.4830408, 3.4830406, 3.4830384, 3.4830394, 3.4830453, 3.4830458, 3.4830437, 3.4830434, 3.4830406, 3.4830427, 3.483044, 3.4830427, 3.4830446, 3.4830432, 3.4830444, 3.4830422, 3.483039, 3.4830413, 3.483046, 3.4830458, 3.4830444, 3.4830413, 3.4830399, 3.4830427, 3.4830434, 3.483044, 3.4830408, 3.4830425, 3.483039, 3.4830475, 3.4830472, 3.4830482, 3.4830446, 3.4830408, 3.4830418, 3.483042, 3.4830375, 3.4830382, 3.4830391, 3.483044, 3.483043, 3.4830403, 3.4830384, 3.4830413, 3.483047, 3.4830372, 3.4830408, 3.483042, 3.483049, 3.4830372, 3.483041, 3.4830368, 3.4830463, 3.4830425, 3.483043, 3.4830441, 3.4830391, 3.4830399, 3.4830377, 3.4830437, 3.48304, 3.4830394, 3.483045, 3.4830418, 3.4830475, 3.4830441, 3.4830446, 3.4830363, 3.483043, 3.483044, 3.483043, 3.4830418, 3.4830391, 3.4830422, 3.4830387, 3.4830444, 3.4830422, 3.483035, 3.483043, 3.4830425, 3.483042, 3.483042, 3.4830356, 3.4830413, 3.4830425, 3.483042, 3.4830441, 3.4830391, 3.483047, 3.4830415, 3.4830403, 3.4830406, 3.4830465, 3.4830444, 3.483038, 3.4830396, 3.483037, 3.4830418, 3.483046, 3.483044, 3.4830456, 3.4830449, 3.4830387, 3.483043, 3.4830484, 3.4830406, 3.4830456, 3.4830403, 3.483044, 3.4830408, 3.4830394, 3.483041, 3.4830434, 3.4830441, 3.4830406, 3.4830406, 3.4830468, 3.483043, 3.4830477, 3.4830415, 3.483044, 3.4830396, 3.483045, 3.4830458, 3.4830472, 3.4830394, 3.4830425, 3.4830449, 3.4830422, 3.4830458, 3.4830406, 3.483042, 3.4830453, 3.483049, 3.4830408, 3.483041, 3.4830406, 3.4830458, 3.4830508, 3.4830399, 3.483039, 3.483042, 3.4830418, 3.4830406, 3.483039, 3.4830458, 3.4830425, 3.4830365, 3.483047, 3.4830418, 3.4830432, 3.4830415, 3.483046, 3.4830406, 3.4830418, 3.4830463, 3.4830434, 3.4830415, 3.4830422, 3.4830437, 3.4830413, 3.4830375, 3.4830425, 3.4830472, 3.4830382, 3.4830372, 3.483038]
  out "Waveform Chart ch2":sgl[](graph)=[3.4783695, 3.4783683, 3.478373, 3.478372, 3.478378, 3.4783747, 3.4783697, 3.4783704, 3.4783719, 3.478371, 3.478373, 3.4783738, 3.478377, 3.4783728, 3.4783702, 3.4783688, 3.478373, 3.4783685, 3.4783714, 3.4783697, 3.4783723, 3.4783728, 3.4783685, 3.4783728, 3.4783733, 3.4783704, 3.4783683, 3.4783728, 3.478367, 3.4783711, 3.4783738, 3.4783747, 3.4783738, 3.4783714, 3.47837, 3.4783652, 3.4783738, 3.4783702, 3.478368, 3.4783766, 3.4783766, 3.478371, 3.4783697, 3.4783752, 3.478371, 3.4783757, 3.47837, 3.4783678, 3.4783723, 3.4783669, 3.4783652, 3.478368, 3.4783702, 3.4783752, 3.4783728, 3.4783745, 3.4783697, 3.4783742, 3.4783754, 3.4783669, 3.4783716, 3.4783654, 3.4783783, 3.4783723, 3.4783695, 3.4783735, 3.4783683, 3.4783669, 3.4783723, 3.478369, 3.478371, 3.4783695, 3.4783707, 3.4783728, 3.4783695, 3.4783714, 3.478368, 3.4783692, 3.4783678, 3.4783669, 3.4783704, 3.4783702, 3.4783695, 3.4783754, 3.4783688, 3.4783697, 3.4783728, 3.4783738, 3.4783683, 3.4783738, 3.478371, 3.4783707, 3.4783745, 3.4783669, 3.478374, 3.4783728, 3.4783728, 3.4783695, 3.4783738, 3.4783685, 3.47837, 3.4783766, 3.478373, 3.4783678, 3.4783711, 3.478367, 3.478368, 3.4783654, 3.478378, 3.4783711, 3.4783714, 3.478366, 3.4783754, 3.4783745, 3.4783716, 3.4783716, 3.4783735, 3.4783704, 3.4783669, 3.4783742, 3.4783745, 3.478372, 3.4783747, 3.4783728, 3.4783697, 3.4783716, 3.4783695, 3.478367, 3.4783747, 3.4783723, 3.4783666, 3.4783738, 3.4783733, 3.4783714, 3.4783735, 3.478374, 3.4783645, 3.4783742, 3.4783664, 3.4783711, 3.478377, 3.4783707, 3.4783692, 3.478372, 3.4783754, 3.4783714, 3.4783683, 3.4783692, 3.4783664, 3.4783728, 3.4783688, 3.4783762, 3.478373, 3.4783707, 3.4783642, 3.4783719, 3.4783735, 3.4783738, 3.4783714, 3.4783754, 3.4783792, 3.4783711, 3.4783716, 3.47837, 3.4783695, 3.478374, 3.4783735, 3.4783733, 3.4783692, 3.4783766, 3.4783735, 3.4783719, 3.4783666, 3.4783654, 3.478371, 3.4783726, 3.4783666, 3.4783719, 3.4783742, 3.478365, 3.478368, 3.4783728, 3.4783697, 3.4783702, 3.478375, 3.4783719, 3.478369, 3.4783697, 3.4783733, 3.478371, 3.4783785, 3.47837, 3.4783735, 3.4783726, 3.4783683, 3.4783697, 3.4783764, 3.478367, 3.47837, 3.4783702]
